vi "Acquire Data.vi"(8 "error in (no error)":errorcluster, 11 "Potentiostat Galvanostat in":refnum<class "Potentiostat Galvanostat.lvclass">) -> (0 "error out":errorcluster, 1 "Channel Data":T1 {"Current Values"."State" items=["Channel is stopped", "Channel is running", "Channel is paused"]; "Current Values"."I Range" items=["I range 100 pA SP-300 series", "I range 1 nA VMP3 / SP-300 series", "I range 10 nA VMP3 / SP-300 series", "I range 100 nA VMP3 / SP-300 series", "I range 1 uA VMP3 / SP-300 series", "I range 10 uA VMP3 / SP-300 series", "I range 100 uA VMP3 / SP-300 series", "I range 1 mA VMP3 / SP-300 series", "I range 10 mA VMP3 / SP-300 series", "I range 100 mA VMP3 / SP-300 series", "I range 1 A VMP3 / SP-300 series", "Booster VMP3 / SP-300 series", "Auto range VMP3 / SP-300 series"]; "Current Values"."Hardware Option Error Code" items=["No Error"=0, "no instrument connected"=-1, "connection in progress"=-2, "selected channel(s) unplugged"=-3, "invalid function parameters"=-4, "selected file does not exist"=-5, "function failed"=-6, "no channel selected"=-7, "invalid instrument configuration"=-8, "EC-Lab firmware loaded on the instrument"=-9, "library not correctly loaded in memory"=-10, "USB library not correctly loaded in memory"=-11, "function of the library already in progress"=-12, "selected channel(s) already used"=-13, "device not allowed"=-14, "Invalid update function parameters"=-15, "internal instrument communication failed"=-101, "too many data to transfer from the instrument (device error)"=-102, "selected channel(s) unplugged (device error)"=-103, "instrument response error"=-104, "invalid message size"=-105]}, 2 "Finished?":bool=TRUE, 3 "Potentiostat Galvanostat out":refnum<class "Potentiostat Galvanostat.lvclass">)   [LabVIEW 2018, in "Potentiostat Galvanostat.lvclass"]
uses:
  Potentiostat Galvanostat.lvclass
  Controls/Channel Data.ctl
  Controls/Process Data.ctl
  Controls/Data Information.ctl
  Controls/Technique ID.ctl
  Controls/Current Values.ctl
  Controls/Channel State.ctl
  Controls/Current Range.ctl
  Controls/Error Codes.ctl
  Potentiostat Galvanostat.lvclass/Potentiostat Galvanostat.ctl
  BL_ConvertNumericIntoSingle.vi
  BL_GetErrorMsg.vi
  <vilib>/Utility/error.llb/Error Cluster From Error Code.vi
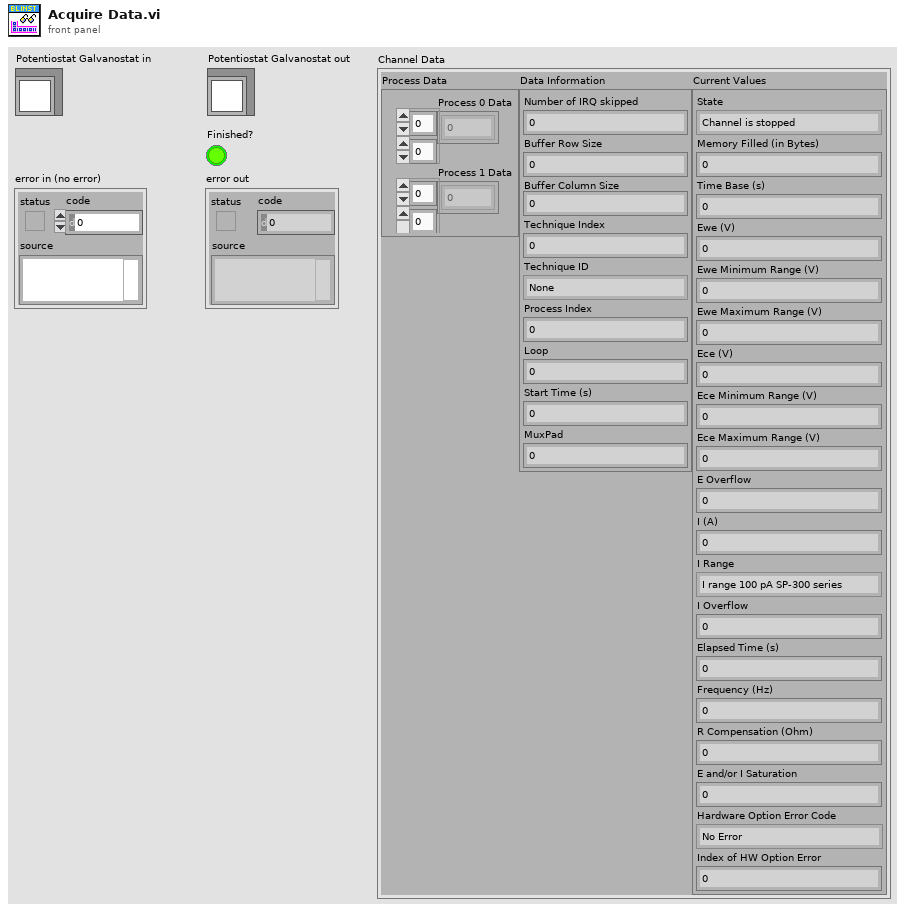
[diagram p1: front panel]
types:
  T1 = typedef "Potentiostat Galvanostat.lvclass/Channel Data.ctl" = cluster{"Process Data":T2, "Data Information":T3, "Current Values":T5}
  T2 = typedef "Potentiostat Galvanostat.lvclass/Process Data.ctl" = cluster{"Process 0 Data":sgl[][], "Process 1 Data":sgl[][]}
  T3 = typedef "Potentiostat Galvanostat.lvclass/Data Information.ctl" = cluster{"Number of IRQ skipped":i32, "Buffer Row Size":i32, "Buffer Column Size":i32, "Technique Index":i32, "Technique ID":T4, "Process Index":i32, "Loop":i32, "Start Time (s)":sgl, "MuxPad":i32}
  T4 = typedef "Potentiostat Galvanostat.lvclass/Technique ID.ctl" = i32
  T5 = typedef "Potentiostat Galvanostat.lvclass/Current Values.ctl" = cluster{"State":T6, "Memory Filled (in Bytes)":i32, "Time Base (s)":sgl, "Ewe (V)":sgl, "Ewe Minimum Range (V)":sgl, "Ewe Maximum Range (V)":sgl, "Ece (V)":sgl, "Ece Minimum Range (V)":sgl, "Ece Maximum Range (V)":sgl, "E Overflow":i32, "I (A)":sgl, "I Range":T7, "I Overflow":i32, "Elapsed Time (s)":dbl, "Frequency (Hz)":sgl, "R Compensation (Ohm)":sgl, "E and/or I Saturation":sgl, "Hardware Option Error Code":T8, "Index of HW Option Error":i32}
  T6 = typedef "Potentiostat Galvanostat.lvclass/Channel State.ctl" = i32
  T7 = typedef "Potentiostat Galvanostat.lvclass/Current Range.ctl" = i32
  T8 = typedef "Potentiostat Galvanostat.lvclass/Error Codes.ctl" = i32
  T9 = typedef "Potentiostat Galvanostat.lvclass/Channel.ctl" = u8
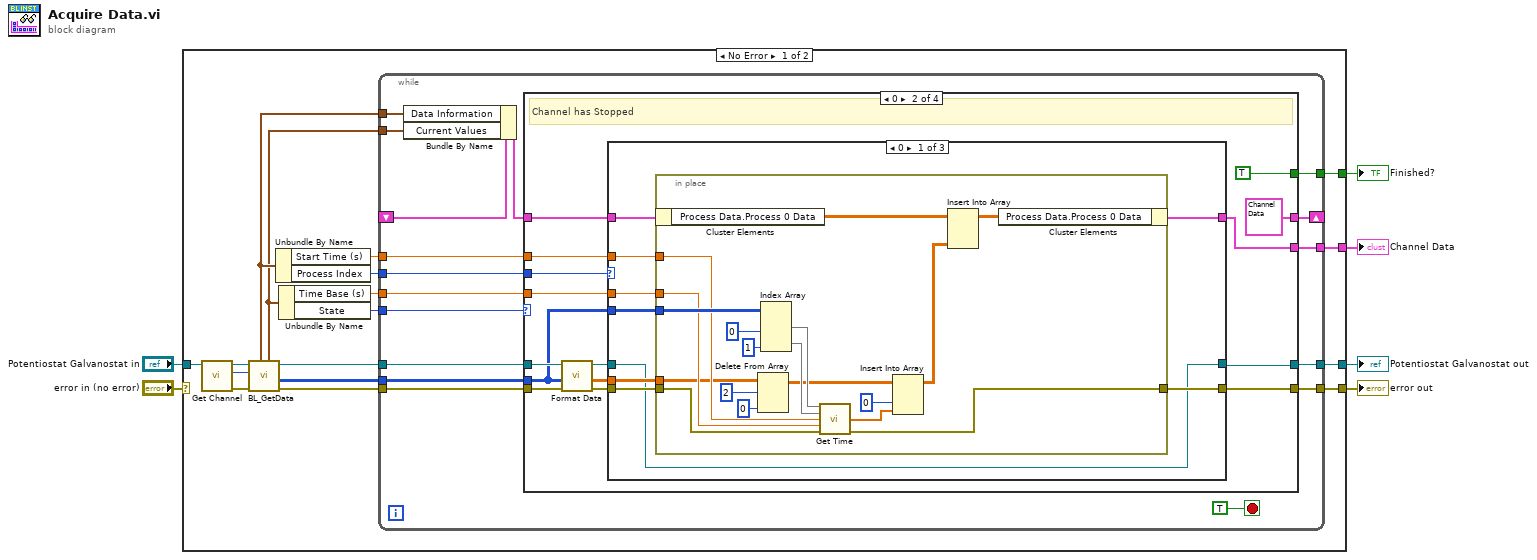
[diagram p0: block diagram]
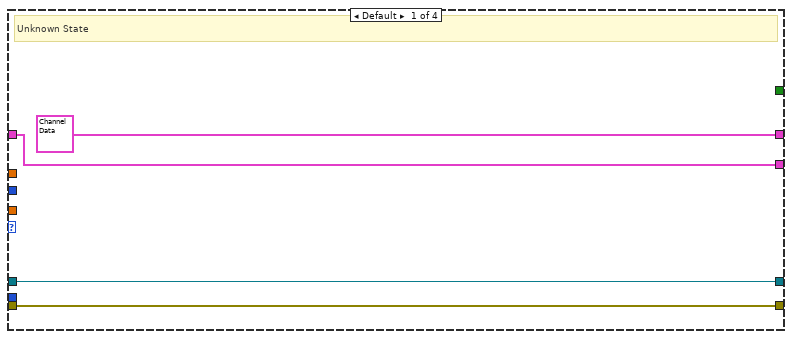
[diagram p2: hidden frame]
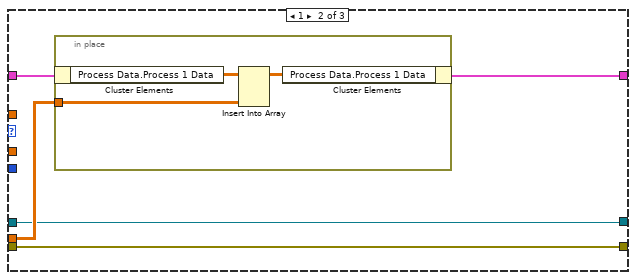
[diagram p3: hidden frame]
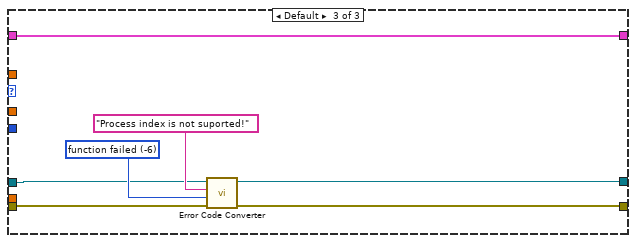
[diagram p4: hidden frame]
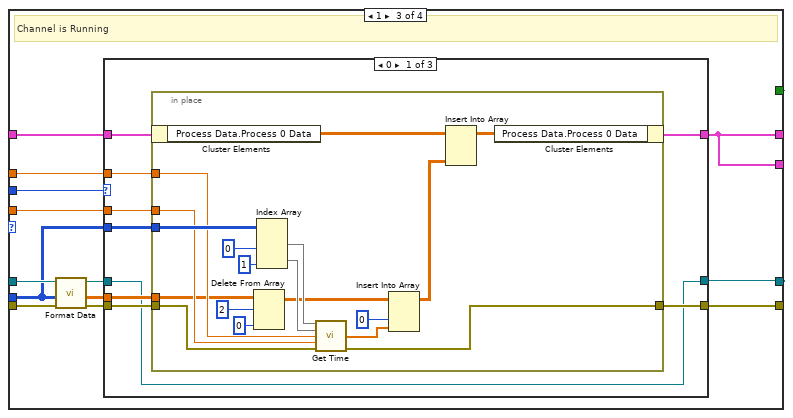
[diagram p5: hidden frame]
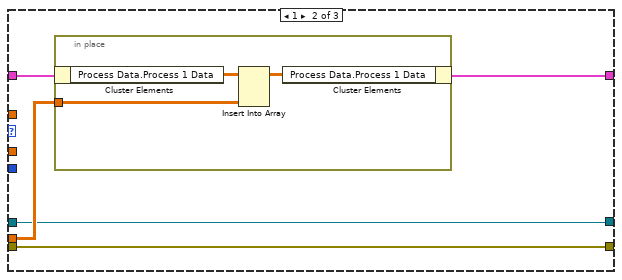
[diagram p6: hidden frame]
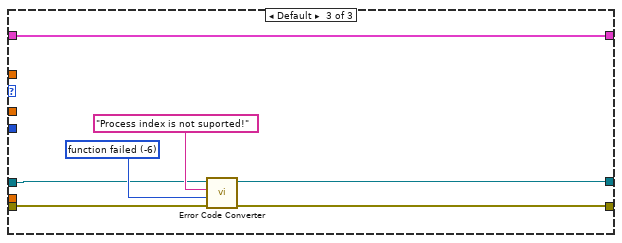
[diagram p7: hidden frame]
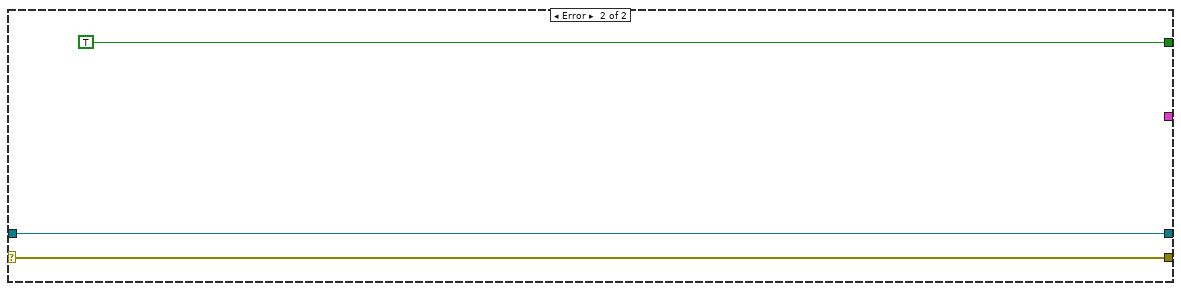
[diagram p9: hidden frame]
diagram:
  n1 = case shown="No Error" "error in (no error)" {
    selector: "error in (no error)" -> [_ w163]
    tunnel: "Potentiostat Galvanostat in" -> [w10 w162]
    tunnel: [w11 w163] -> w4
    tunnel: [w8 w162] -> w3
    tunnel: [w9 TRUE] -> w2
    tunnel: [w7 _] -> w1
    frame No Error {
      n2 = call "Get Channel.vi"("Potentiostat Galvanostat in"=w10) -> ("error out"=w22:errorcluster, "Channel"=w21:T9, "Potentiostat Galvanostat out"=w23:refnum<class "Potentiostat Galvanostat.lvclass">)  [unwired: 8 in]
      n3 = call "BL_GetData.vi"("error in (no error)"=w22, "Channel"=w21, "Potentiostat Galvanostat in"=w23) -> ("error out"=w20:errorcluster, "Data Buffer"=w14:u32[][], "Potentiostat Galvanostat out"=w19:refnum<class "Potentiostat Galvanostat.lvclass">, "Current Values"=w12:T5, "Data Information"=w13:T3)  [unwired: 3 in, 1 out]
      n4 = Unbundle By Name(w13) -> ("Start Time (s)"=w15:sgl, "Process Index"=w16:i32)
      n5 = Unbundle By Name(w12) -> ("Time Base (s)"=w17:sgl, "State"=w18:T6)
      n6 = while {
        tunnel: w20 -> [w39]
        tunnel: w19 -> [w40]
        tunnel: w18 -> [w26]
        tunnel: w17 -> [w38]
        tunnel: w16 -> [w37]
        tunnel: w15 -> [w36]
        tunnel: w14 -> [w35]
        tunnel: w13 -> [w27]
        tunnel: w12 -> [w28]
        shift-right: [w34] -> _
        shift-left: _ -> [w25]
        tunnel: [w33] -> w11
        tunnel: [w31] -> w9
        tunnel: [w30] -> w8
        tunnel: [w24] -> w7
        stop <- TRUE stop-if-true
        n7 = Bundle By Name(cluster=w25, "Data Information"=w27, "Current Values"=w28) -> (w29:T1)
        n8 = case shown="0" w26 {
          tunnel: w40 -> [w42 w49 w114 w159]
          tunnel: w39 -> [w41 w54 w115 w160]
          tunnel: w38 -> [_ w53 w111 _]
          tunnel: w37 -> [_ w52 w113 _]
          tunnel: w36 -> [_ w51 w112 _]
          tunnel: w35 -> [_ w48 w109 _]
          tunnel: [T1 {"Process Data"={"Process 0 Data"=[], "Process 1 Data"=[]}, "Data Information"={"Number of IRQ skipped"=0, "Buffer Row Size"=0, "Buffer Column Size"=0, "Technique Index"=0, "Technique ID"=0, "Process Index"=0, "Loop"=0, "Start Time (s)"=0.0, "MuxPad"=0}, "Current Values"={"State"=0, "Memory Filled (in Bytes)"=0, "Time Base (s)"=0.0, "Ewe (V)"=0.0, "Ewe Minimum Range (V)"=0.0, "Ewe Maximum Range (V)"=0.0, "Ece (V)"=0.0, "Ece Minimum Range (V)"=0.0, "Ece Maximum Range (V)"=0.0, "E Overflow"=0, "I (A)"=0.0, "I Range"=0, "I Overflow"=0, "Elapsed Time (s)"=0.0, "Frequency (Hz)"=0.0, "R Compensation (Ohm)"=0.0, "E and/or I Saturation"=0.0, "Hardware Option Error Code"=0, "Index of HW Option Error"=0}} ("Data Channel") T1 {"Process Data"={"Process 0 Data"=[], "Process 1 Data"=[]}, "Data Information"={"Number of IRQ skipped"=0, "Buffer Row Size"=0, "Buffer Column Size"=0, "Technique Index"=0, "Technique ID"=0, "Process Index"=0, "Loop"=0, "Start Time (s)"=0.0, "MuxPad"=0}, "Current Values"={"State"=0, "Memory Filled (in Bytes)"=0, "Time Base (s)"=0.0, "Ewe (V)"=0.0, "Ewe Minimum Range (V)"=0.0, "Ewe Maximum Range (V)"=0.0, "Ece (V)"=0.0, "Ece Minimum Range (V)"=0.0, "Ece Maximum Range (V)"=0.0, "E Overflow"=0, "I (A)"=0.0, "I Range"=0, "I Overflow"=0, "Elapsed Time (s)"=0.0, "Frequency (Hz)"=0.0, "R Compensation (Ohm)"=0.0, "E and/or I Saturation"=0.0, "Hardware Option Error Code"=0, "Index of HW Option Error"=0}} ("Data Channel") w102 w158] -> w34
          tunnel: w29 -> [w43 w50 w110 w158]
          tunnel: [w41 w47 w106 w160] -> w33
          tunnel: [_ TRUE FALSE _] -> w31
          tunnel: [w42 w46 w104 w159] -> w30
          tunnel: [w43 w45 w102 w158] -> w24
          frame Default {
            # "Unknown State"
          }
          frame 0 {
            # "Channel has Stopped"
            n9 = call "Format Data.vi"("error in (no error)"=w54, "Data Buffer"=w48, "Potentiostat Galvanostat in"=w49) -> ("error out"=w56:errorcluster, "Data"=w57:sgl[][], "Potentiostat Galvanostat out"=w55:refnum<class "Potentiostat Galvanostat.lvclass">)  [unwired: 6 in]
            n10 = case shown="0" w52 {
              tunnel: w51 -> [w65 _ _]
              tunnel: w53 -> [w66 _ _]
              tunnel: [w60 w87 w95] -> w45
              tunnel: w50 -> [w61 w88 w95]
              tunnel: w48 -> [w67 _ _]
              tunnel: w57 -> [w64 w91 _]
              tunnel: w56 -> [w68 w90 w98]
              tunnel: [w63 w90 w97] -> w47
              tunnel: w55 -> [w62 w89 w99]
              tunnel: [w62 w89 w96] -> w46
              frame 0 {
                n11 = in-place {
                  in-place-border: w68 -> [w86]
                  in-place-border: w67 -> [w83]
                  in-place-border: w66 -> [w82]
                  in-place-border: w65 -> [w81]
                  in-place-border: w64 -> [w77]
                  in-place-border: [w71] -> w63
                  n12 = in-place-cluster #1(w61) -> ("Process Data.Process 0 Data"=w70:sgl[][])
                  n13 = Delete From Array(array=w77, length=2, index (col)=0 ("disabled index (col)")) -> (array with subset deleted=w74:sgl[][])  [unwired: 1 in, 1 out]
                  n14 = Index Array(array=w83, index (col) #1=0 ("disabled index (col)"), index (col) #2=1 ("index (col)")) -> (element #1=w76:u32[], element #2=w80:u32[])  [unwired: 2 in]
                  n15 = call "Get Time.vi"("t_high"=w76, "t_low"=w80, "Start Time (s)"=w81, "Time Base (s)"=w82, "error in (no error)"=w86) -> ("Time"=w73:dbl[], "error out"=w71:errorcluster)  [unwired: 9 in]
                  n16 = Insert Into Array(array=w74, index (col)=0 ("disabled index (col)"), new element=w73) -> (w72:sgl[][])  [unwired: 1 in]
                  n17 = Insert Into Array(array=w70, new element=w72) -> (w69:sgl[][])  [unwired: 2 in]
                  n18 = in-place-cluster #1("Process Data.Process 0 Data"=w69) -> (w60:T1)
                }
              }
              frame 1 {
                n19 = in-place {
                  in-place-border: w91 -> [w94]
                  n20 = in-place-cluster #2(w88) -> ("Process Data.Process 1 Data"=w93:sgl[][])
                  n21 = Insert Into Array(array=w93, new element=w94) -> (w92:sgl[][])  [unwired: 2 in]
                  n22 = in-place-cluster #2("Process Data.Process 1 Data"=w92) -> (w87:T1)
                }
              }
              frame Default {
                w101 = T8 -6 items=["No Error"=0, "no instrument connected"=-1, "connection in progress"=-2, "selected channel(s) unplugged"=-3, "invalid function parameters"=-4, "selected file does not exist"=-5, "function failed"=-6, "no channel selected"=-7, "invalid instrument configuration"=-8, "EC-Lab firmware loaded on the instrument"=-9, "library not correctly loaded in memory"=-10, "USB library not correctly loaded in memory"=-11, "function of the library already in progress"=-12, "selected channel(s) already used"=-13, "device not allowed"=-14, "Invalid update function parameters"=-15, "internal instrument communication failed"=-101, "too many data to transfer from the instrument (device error)"=-102, "selected channel(s) unplugged (device error)"=-103, "instrument response error"=-104, "invalid message size"=-105] ("Error Code")
                n23 = call "Error Code Converter.vi"("error in (no error)"=w98, "Error Code"=w101, "Additional Description"="Process index is not suported!", "Potentiostat Galvanostat in"=w99) -> ("error out"=w97:errorcluster, "Potentiostat Galvanostat out"=w96:refnum<class "Potentiostat Galvanostat.lvclass">)  [unwired: 6 in]
              }
            }
          }
          frame 1 {
            # "Channel is Running"
            n24 = call "Format Data.vi"("error in (no error)"=w115, "Data Buffer"=w109, "Potentiostat Galvanostat in"=w114) -> ("error out"=w107:errorcluster, "Data"=w108:sgl[][], "Potentiostat Galvanostat out"=w105:refnum<class "Potentiostat Galvanostat.lvclass">)  [unwired: 6 in]
            n25 = case shown="0" w113 {
              tunnel: w112 -> [w121 _ _]
              tunnel: w111 -> [w122 _ _]
              tunnel: [w116 w143 w151] -> w102
              tunnel: w110 -> [w117 w144 w151]
              tunnel: w109 -> [w123 _ _]
              tunnel: w108 -> [w120 w147 _]
              tunnel: w107 -> [w124 w146 w154]
              tunnel: [w119 w146 w153] -> w106
              tunnel: w105 -> [w118 w145 w155]
              tunnel: [w118 w145 w152] -> w104
              frame 0 {
                n26 = in-place {
                  in-place-border: w124 -> [w142]
                  in-place-border: w123 -> [w139]
                  in-place-border: w122 -> [w138]
                  in-place-border: w121 -> [w137]
                  in-place-border: w120 -> [w133]
                  in-place-border: [w127] -> w119
                  n27 = in-place-cluster #3(w117) -> ("Process Data.Process 0 Data"=w126:sgl[][])
                  n28 = Delete From Array(array=w133, length=2, index (col)=0 ("disabled index (col)")) -> (array with subset deleted=w130:sgl[][])  [unwired: 1 in, 1 out]
                  n29 = Index Array(array=w139, index (col) #1=0 ("disabled index (col)"), index (col) #2=1 ("index (col)")) -> (element #1=w132:u32[], element #2=w136:u32[])  [unwired: 2 in]
                  n30 = call "Get Time.vi"("t_high"=w132, "t_low"=w136, "Start Time (s)"=w137, "Time Base (s)"=w138, "error in (no error)"=w142) -> ("Time"=w129:dbl[], "error out"=w127:errorcluster)  [unwired: 9 in]
                  n31 = Insert Into Array(array=w130, index (col)=0 ("disabled index (col)"), new element=w129) -> (w128:sgl[][])  [unwired: 1 in]
                  n32 = Insert Into Array(array=w126, new element=w128) -> (w125:sgl[][])  [unwired: 2 in]
                  n33 = in-place-cluster #3("Process Data.Process 0 Data"=w125) -> (w116:T1)
                }
              }
              frame 1 {
                n34 = in-place {
                  in-place-border: w147 -> [w150]
                  n35 = in-place-cluster #4(w144) -> ("Process Data.Process 1 Data"=w149:sgl[][])
                  n36 = Insert Into Array(array=w149, new element=w150) -> (w148:sgl[][])  [unwired: 2 in]
                  n37 = in-place-cluster #4("Process Data.Process 1 Data"=w148) -> (w143:T1)
                }
              }
              frame Default {
                w157 = T8 -6 items=["No Error"=0, "no instrument connected"=-1, "connection in progress"=-2, "selected channel(s) unplugged"=-3, "invalid function parameters"=-4, "selected file does not exist"=-5, "function failed"=-6, "no channel selected"=-7, "invalid instrument configuration"=-8, "EC-Lab firmware loaded on the instrument"=-9, "library not correctly loaded in memory"=-10, "USB library not correctly loaded in memory"=-11, "function of the library already in progress"=-12, "selected channel(s) already used"=-13, "device not allowed"=-14, "Invalid update function parameters"=-15, "internal instrument communication failed"=-101, "too many data to transfer from the instrument (device error)"=-102, "selected channel(s) unplugged (device error)"=-103, "instrument response error"=-104, "invalid message size"=-105] ("Error Code")
                n38 = call "Error Code Converter.vi"("error in (no error)"=w154, "Error Code"=w157, "Additional Description"="Process index is not suported!", "Potentiostat Galvanostat in"=w155) -> ("error out"=w153:errorcluster, "Potentiostat Galvanostat out"=w152:refnum<class "Potentiostat Galvanostat.lvclass">)  [unwired: 6 in]
              }
            }
          }
          frame 2 {
            # "Channel is paused"
          }
        }
      }
    }
    frame Error {
    }
  }
  "error out" <- w4
  "Potentiostat Galvanostat out" <- w3
  "Channel Data" <- w1
  "Finished?" <- w2
